vi "Init and Rotate array Double.vi"(5 "Reset":bool, 7 "Stop read":bool, 9 "Array size":i32=30, 11 "PV":dbl) -> (3 "Array":dbl[](array[numeric]))   [LabVIEW 2019, in "Userlib.lvlib"]
uses:
  Userlib.lvlib
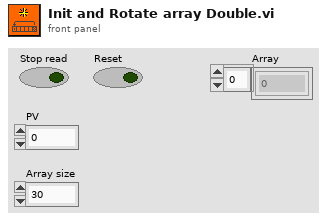
[diagram p1: front panel]
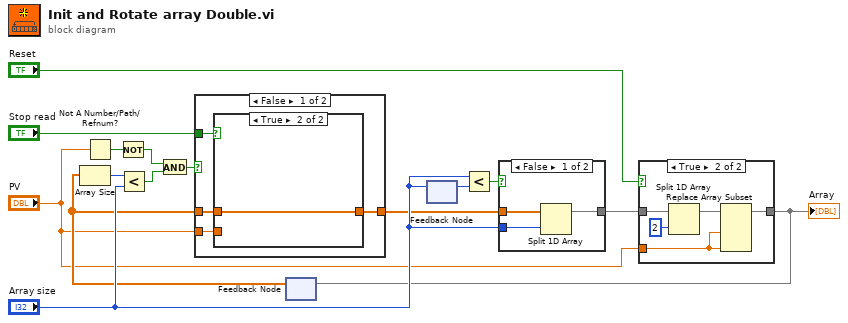
[diagram p0: block diagram]
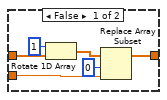
[diagram p3: hidden frame]
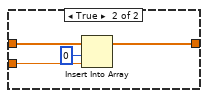
[diagram p4: hidden frame]
diagram:
  n1 = Not A Number/Path/Refnum?(number/path/refnum="PV") -> (NaN/Path/Refnum?=w9:bool)
  n2 = Not(x=w9) -> (.not. x?=w8:bool)
  n3 = feedback #1() -> (w12:dbl[])  [unwired: 1 in]
  n4 = Array Size(array=w12) -> (size(s)=w13:i32)
  n5 = Less?(x=w13, y="Array size") -> (x < y?=w11:bool)
  n6 = And(x=w8, y=w11) -> (x .and. y?=w10:bool)
  n7 = case shown="False" w10 {
    tunnel: [w17 w30] -> w7
    tunnel: "PV" -> [w18 w27]
    tunnel: w12 -> [w19 w29]
    tunnel: "Stop read" -> [w16 _]
    frame False {
      n8 = case shown="True" w16 {
        tunnel: w19 -> [w22 w26]
        tunnel: w18 -> [w21 _]
        tunnel: [w20 w26] -> w17
        frame False {
          n9 = Rotate 1D Array(1:w22, 2:1 ("n")) -> (0:w24:dbl[])
          n10 = Replace Array Subset(array=w24, new element=w21, index=0) -> (w20:dbl[])
        }
        frame True {
        }
      }
    }
    frame True {
      n11 = Insert Into Array(array=w29, index=0, new element=w27) -> (w30:dbl[])
    }
  }
  n12 = feedback #2() -> (w6:i32)  [unwired: 1 in]
  n13 = feedback-in #2("Array size") -> ()
  n14 = Less?(x="Array size", y=w6) -> (x < y?=w5:bool)
  n15 = case shown="False" w5 {
    tunnel: [w31 w34] -> w4
    tunnel: w7 -> [w33 w34]
    tunnel: "Array size" -> [w32 _]
    frame False {
      n16 = Split 1D Array(array=w33, index=w32) -> (first subarray=w31:dbl[])  [unwired: 1 out]
    }
    frame True {
    }
  }
  n17 = case shown="True" "Reset" {
    tunnel: [w35 w37] -> w1
    tunnel: w4 -> [w35 w40]
    tunnel: "PV" -> [_ w36]
    frame False {
    }
    frame True {
      n18 = Split 1D Array(array=w40, index=2) -> (first subarray=w39:dbl[])  [unwired: 1 out]
      n19 = Replace Array Subset(array=w39, new element #1=w36, new element #2=w36) -> (w37:dbl[])  [unwired: 2 in]
    }
  }
  "Array" <- w1
  n20 = feedback-in #1(w1) -> ()
